vi "PH_OceanOpticsSpectrometer.Set Integration Time.vi"(0 "i ref in":refnum<vi>, 5 "error in (no error)":errorcluster) -> (14 "i ref out":refnum<vi>, 19 "error out":errorcluster)   [LabVIEW 2014, in "PH_OceanOpticsSpectrometer.lvlib"]
doc: "This VI sets the integration time."
uses:
  PH_OceanOpticsSpectrometer.lvlib
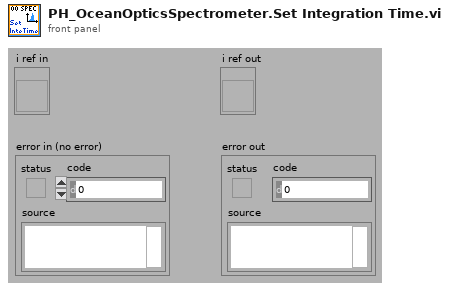
[diagram p1: front panel]
types:
  T1 = typedef "PH_OceanOpticsSpectrometer.lvlib/PH_OceanOpticsSpectrometer.i attribute.ctl" = cluster{"GUI Refs":cluster{"Delete":refnum<vi>, "Spectrum":refnum<vi>, "Display Width":refnum<vi>, "Display Center":refnum<vi>, "Save":refnum<vi>, "Integration time":refnum<vi>, "center wavelength":refnum<vi>, "width":refnum<vi>, "Wanted Trigger Mode":refnum<vi>, "Current Trigger Mode":refnum<vi>, "Trigger Info":refnum<vi>, "Model":refnum<vi>, "Driver":refnum<vi>, "Firmware":refnum<vi>}, "Display":cluster{"Width":dbl, "Center":dbl}, "VISA resource name":refnum<visa-resource-name>, "Integration time [ms]":cluster{"Current Value":u16, "Wanted Value":u16}, "Trigger":cluster{"Current value":T2, "Wanted value":T2}, "Default VISA Timeout":u32, "Last Data":cluster{"Wavelength Bins":dbl[], "Spectrum by Pixels":dbl[]}}
  T2 = typedef "PH_OceanOpticsSpectrometer.lvlib/PH_OceanOpticsSpectrometer.Trigger.ctl" = enum32{"External", "Normal"}
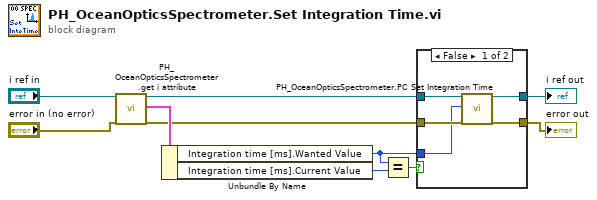
[diagram p0: block diagram]
diagram:
  n1 = call "PH_OceanOpticsSpectrometer.get i attribute.vi"("i ref in"="i ref in", "error in (no error)"="error in (no error)") -> ("i ref out"=w2:refnum<vi>, "i attribute"=w10:T1, "error out"=w1:errorcluster)  [unwired: 15 in]
  n2 = Unbundle By Name(w10) -> ("Integration time [ms].Wanted Value"=w3:u16, "Integration time [ms].Current Value"=w5:u16)
  n3 = Equal?(x=w3, y=w5) -> (x = y?=w4:bool)
  n4 = case shown="False" w4 {
    tunnel: [w15 w17] -> w9
    tunnel: [w14 w16] -> w7
    tunnel: w2 -> [w13 w16]
    tunnel: w1 -> [w12 w17]
    tunnel: w3 -> [w11 _]
    frame False {
      n5 = call "PH_OceanOpticsSpectrometer.PC Set Integration Time.vi"("VI in"=w13, "Wanted Integration Time [ms]"=w11, "error in (no error)"=w12) -> ("VI out"=w14:refnum<vi>, "error out"=w15:errorcluster)  [unwired: 15 in]
    }
    frame True {
    }
  }
  "error out" <- w9
  "i ref out" <- w7
